vi "Queue to Name.vi"(0 "Queue in":refnum<queue>) -> (5 "Found?":bool, 6 "Queue Name out":string)   [LabVIEW 2021, in "Queue.lvlib"]
uses:
  Queue.lvlib
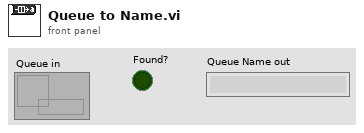
[diagram p1: front panel]
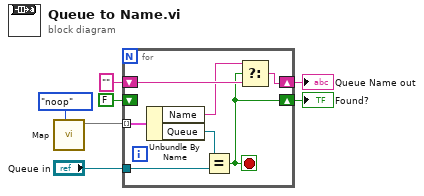
[diagram p0: block diagram]
diagram:
  n1 = call "Map.vi"("Action"=enum8{"noop", "get", "set", "pop"}."noop") -> ("Queue Map"=w6:map{string, refnum<queue>})  [unwired: 8 in, 2 out]
  n2 = for {
    tunnel: w6 -> [w14] mode=indexing
    tunnel: "Queue in" -> [w12]
    shift-right: [w9] -> w3
    shift-left: "" ("Name") -> [w11]
    shift-right: [w8] -> w1
    shift-left: FALSE -> [_]
    stop <- w8 stop-if-true
    n3 = Unbundle By Name(w14) -> ("Name"=w10:string, "Queue"=w13:refnum<queue>)
    n4 = Equal?(x=w13, y=w12) -> (x = y?=w8:bool)
    n5 = Select(t=w10, s=w8, f=w11) -> (s? t:f=w9:string)
  }
  "Queue Name out" <- w3
  "Found?" <- w1
